vi "List Keys.vi"(8 "error in (no error)":errorcluster, 10 "Section Name":string, 11 "CSM-Static-Variable-Manager in":refnum<class "CSM-Static-Variable-Manager.lvclass">) -> (0 "error out":errorcluster, 1 "Array":string[](array[string]), 2 "Key?":bool, 3 "CSM-Static-Variable-Manager out":refnum<class "CSM-Static-Variable-Manager.lvclass">)   [LabVIEW 2017, in "INI-Static-Variable-Support.lvlib" / "CSM-Static-Variable-Manager.lvclass"]
uses:
  CSM-Static-Variable-Manager.lvclass
  CSM-Static-Variable-Manager.lvclass/CSM-Static-Variable-Manager.ctl
  LabVIEW-Config/LabVIEW-Config.lvclass
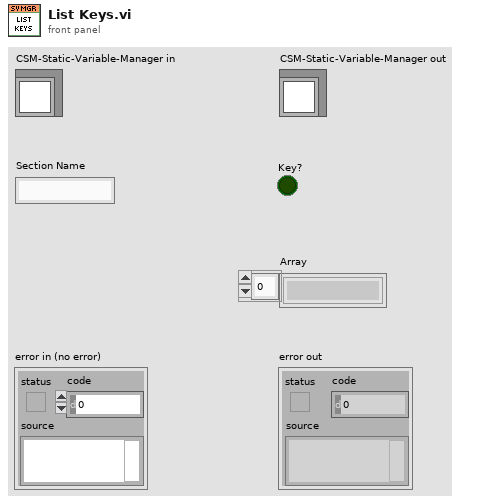
[diagram p1: front panel]
types:
  T1 = typedef "LabVIEW-Config.lvlib/Config.ctl" = cluster{"Path":path, "Lines":string[], "Tokens":T2[], "Modified?":bool, "Cache":cluster{"Valid?":bool, "Key Information":T3[]}}
  T2 = typedef "LabVIEW-Config.lvlib/LineToken.ctl" = enum8{"comment", "section", "key", "more"}
  T3 = typedef "LabVIEW-Config.lvlib/KeyInfo.ctl" = cluster{"Key Indexes":cluster{"Indexes":i32[]}[], "Session Found?":bool, "Key found?":bool, "Session Index":i32}
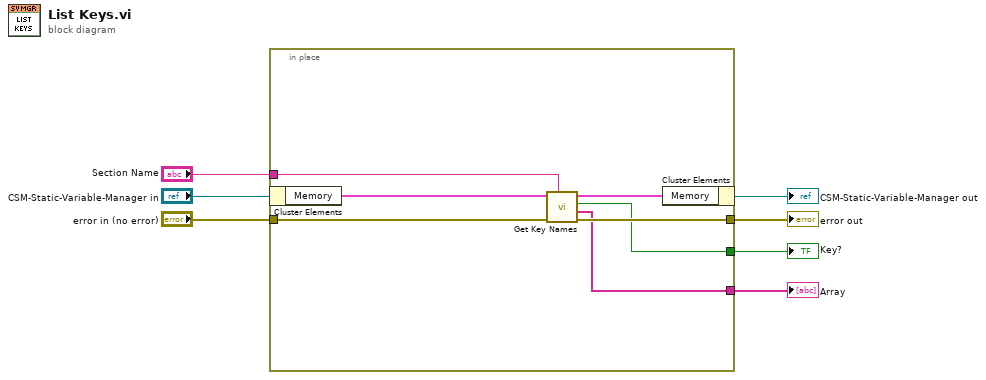
[diagram p0: block diagram]
diagram:
  n1 = in-place {
    in-place-border: "Section Name" -> [w12]
    in-place-border: "error in (no error)" -> [w11]
    in-place-border: [w10] -> w3
    in-place-border: [w9] -> w2
    in-place-border: [w8] -> w1
    n2 = in-place-cluster #1("CSM-Static-Variable-Manager in") -> ("Memory"=w14:T1)
    n3 = call "Get Key Names.vi"("Section Name"=w12, "error in (no error)"=w11, "Config in"=w14) -> ("error out"=w10:errorcluster, "Key Names"=w9:string[], "Section Found?"=w8:bool, "Config out"=w13:T1)  [unwired: 5 in]
    n4 = in-place-cluster #1("Memory"=w13) -> (→"CSM-Static-Variable-Manager out":refnum<class "CSM-Static-Variable-Manager.lvclass">)
  }
  "error out" <- w3
  "Array" <- w2
  "Key?" <- w1
